vi "ATF-Disconnect RT.vi"(8 "error in (no error)":errorcluster, 10 "RT Disconnect":enum16{"Both", "Pump", "Storage"}(ring), 11 "Cluster in":T3) -> (0 "error out":errorcluster, 2 "status":string, 3 "Cluster out":T3)   [LabVIEW 2022 SP3]
uses:
  Controls/SeCrTs-boolean ref.ctl
  Controls/SeCrTs-EPV .ctl
  75c43d07-cfec-4a61-aeb0-3d2073dd9aa1.vi
  ebca87ca-1d58-4613-b13f-b88391691f9b.vi
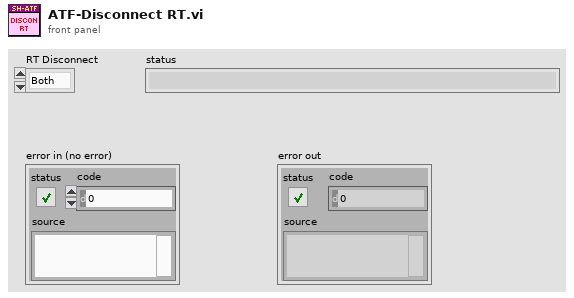
[diagram p1: front panel]
types:
  T1 = typedef "SeCrTs-boolean ref.ctl" = cluster{"Connect RT":refnum<vi>, "START DAQ":refnum<vi>, "STOP DAQ":refnum<vi>, "DAQ SETTING":refnum<vi>, "START LOG":refnum<vi>, "STOP LOG":refnum<vi>, "Connect Drive ATF":refnum<vi>, "Update drive ATF":refnum<vi>, "Gate driver ATF":refnum<vi>, "Motor On ATF":refnum<vi>, "ADC reset ATF":refnum<vi>, "Gate driver ATF 2":refnum<vi>, "Motor off ATF":refnum<vi>, "MCU reset ATF":refnum<vi>, "Connect Drive Lox":refnum<vi>, "Update drive lox":refnum<vi>, "Gate driver- LOX":refnum<vi>, "Motor On lox":refnum<vi>, "Adc reset lox":refnum<vi>, "MCU Reset -LOX":refnum<vi>, "Motor Off lox":refnum<vi>, "Connect ppsu":refnum<vi>, "update ppsu":refnum<vi>, "DC on":refnum<vi>, "Alarm ack":refnum<vi>, "DC off":refnum<vi>, "Ms initialize":refnum<vi>, "Exit RT":refnum<vi>, "ABORT":refnum<vi>, "HOLD UPDATE":refnum<vi>, "Log type":refnum<vi>, "PUMP IP":refnum<vi>, "STORAGE IP":refnum<vi>}
  T2 = typedef "SeCrTs-EPV .ctl" = cluster{"F_EPV_131":refnum<vi>, "F_EPV_132":refnum<vi>, "F_EPV_136":refnum<vi>, "F_EPV_21":refnum<vi>, "F_EPV_41":refnum<vi>, "N_EPV_68":refnum<vi>, "N_EPV_ 69":refnum<vi>, "N_EPV_ 33":refnum<vi>, "F_EPV_142":refnum<vi>, "F_EPV_28":refnum<vi>, "N_EPV_203":refnum<vi>, "N_EPV_206":refnum<vi>, "F_EPV_75":refnum<vi>, "C_EPV_2":refnum<vi>, "C_EPV_7":refnum<vi>, "C_EPV_8":refnum<vi>, "C_EPV_123":refnum<vi>, "C_EPV_124":refnum<vi>, "C_EPV_127":refnum<vi>, "N_EPV_62a":refnum<vi>, "N_EPV_62b":refnum<vi>, "N_EPV_61":refnum<vi>, "G_EPV_51":refnum<vi>, "N_EPV_141":refnum<vi>, "C_EPV_803":refnum<vi>, "C_EPV_18":refnum<vi>, "C_EPV_1352":refnum<vi>, "N_EPV_202":refnum<vi>, "C_EPV_16":refnum<vi>}
  T3 = cluster{"Bol":T1, "EPV":T2, "Covers":cluster{"cover":refnum<vi>, "Login screen cover":refnum<vi>, "cover Motor":refnum<vi>}, "Log cmd":cluster{"C/NC":bool, "Start/Stop Log":bool[], "Log Name":string, "Config":cluster{"AO config":cluster{"Channel_Name":string, "Channel_Number":string, "Default_Value":dbl, "Units":string}[], "AI config":cluster{"Channel_Name":string, "Channel_Number":string, "Pre_Scale_min":dbl, "Pre_Scale_max":dbl, "Sensor_min":dbl, "Sensor_max":dbl, "Units":string}[], "DI config":cluster{"Channel_Name":string, "Channel_Number":string, "Default_Value":bool, "DI invert?":bool}[], "DO config":cluster{"Channel_Name":string, "Channel_Number":string, "Default_Value":bool, "DO invert?":bool}[], "TC config":cluster{"Channel_Name":string, "Channel_Number":string, "Pre_Scale_min":dbl, "Pre_Scale_max":dbl, "units":i32, " type":i32}[], "ACC config":cluster{"Channel_Name":string, "Channel_Number":string, "Pre_Scale_min":dbl, "Pre_Scale_max":dbl, "Terminal configuration":i32, "Sensitivity":dbl, "Sensitivity units":i32}[], "SG config":cluster{"Channel_Name":string, "Channel_Number":string, "Pre_Scale_min":dbl, "Pre_Scale_max":dbl}[], "Strain Gauge Settings":cluster{"poisson ratio":dbl, "nominal gage resistance":dbl, "gage factor":dbl}, "Bridge Settings":cluster{"voltage excitation value":dbl, "voltage excitation source":i32, "initial bridge voltage":dbl, "lead wire resistance":dbl, "strain configuration":i32}, "Sample Rate":cluster{"AI Sample Rate":dbl[], "AO Sample Rate":dbl[], "DI Sample Rate":dbl[], "TC Sample Rate":dbl[], "DO Sample Rate":dbl[], "SG Sample Rate":dbl[], "ACC Sample Rate":dbl[]}}, "Log min":dbl}, "STORAGE IP":string, "PUMP IP":string, "Storage con":bool, "Pumb con":bool}
  T4 = enum8{"Enabled", "Disabled", "Disabled and Grayed Out"}
  T5 = enum8{"Enabled", "Disabled", "Disabled and Grayed Out"}[]
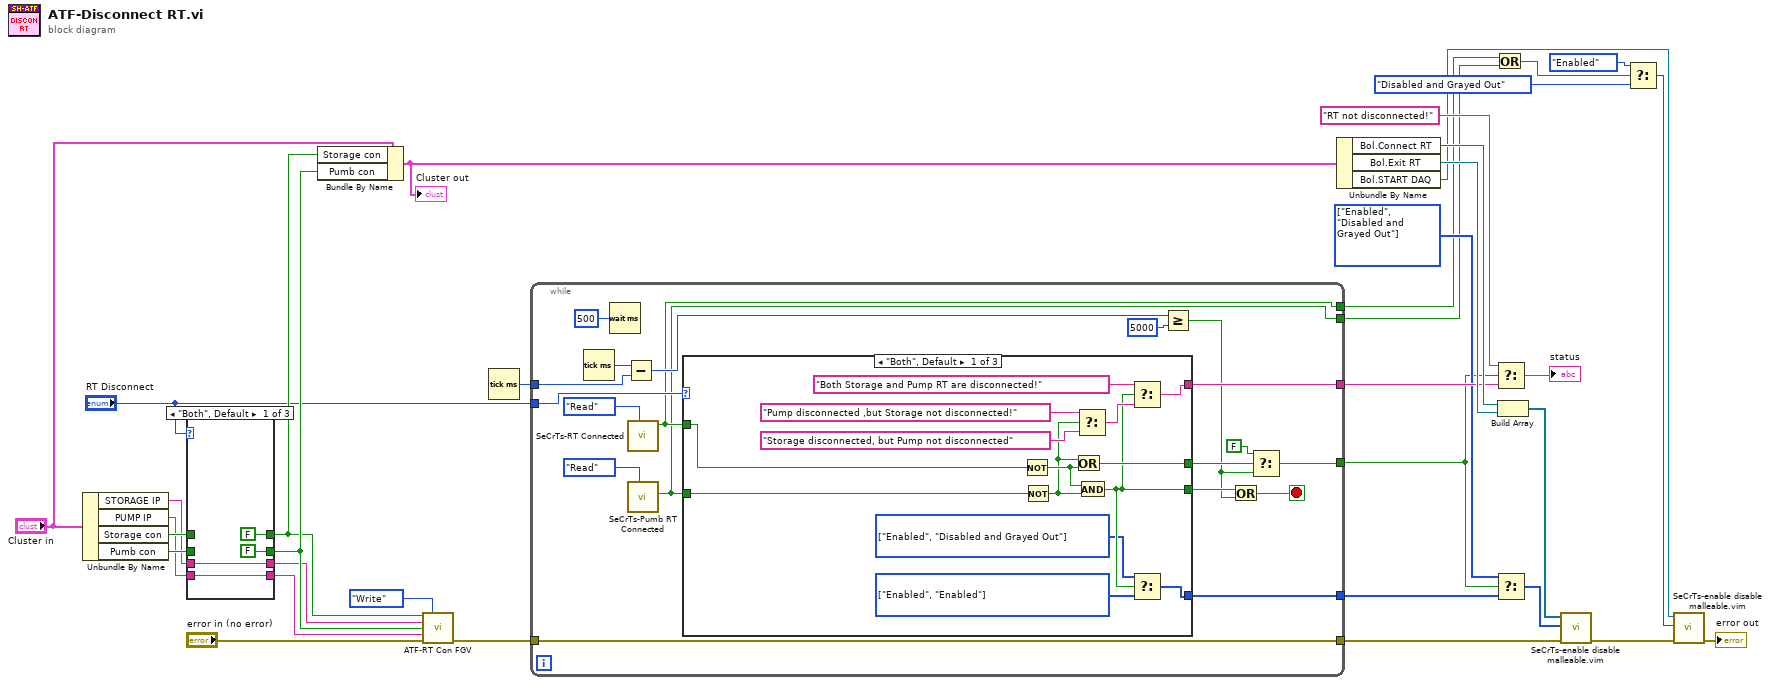
[diagram p0: block diagram]
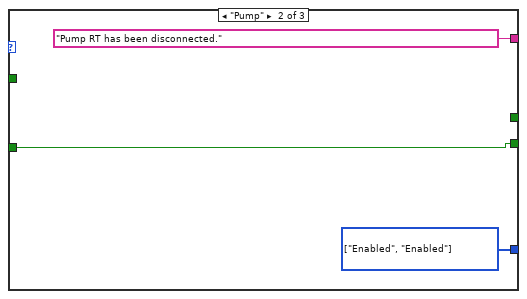
[diagram p2: hidden frame]
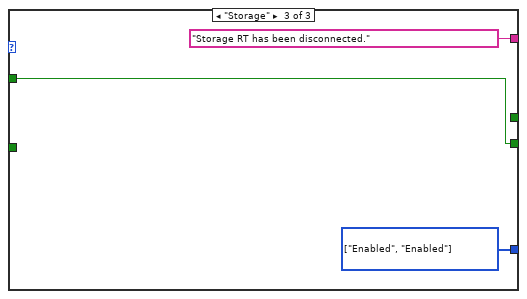
[diagram p3: hidden frame]
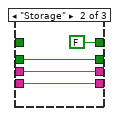
[diagram p4: hidden frame]
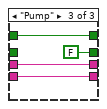
[diagram p5: hidden frame]
diagram:
  w17 = T5 [enum."Enabled", enum."Disabled and Grayed Out"] items=["Enabled", "Disabled", "Disabled and Grayed Out"] ("t")
  n1 = Unbundle By Name("Cluster in") -> ("STORAGE IP"=w30:string, "PUMP IP"=w31:string, "Storage con"=w32:bool, "Pumb con"=w33:bool)
  n2 = case shown="\"Both\", Default" "RT Disconnect" {
    tunnel: [w37 w42 w47] -> w27
    tunnel: [FALSE ("Storage rt con") FALSE ("Storage rt con") w44] -> w34
    tunnel: w30 -> [w37 w42 w47]
    tunnel: w31 -> [w36 w41 w46]
    tunnel: [w36 w41 w46] -> w29
    tunnel: [FALSE ("Pumb rt con") w40 FALSE ("Pumb rt con")] -> w35
    tunnel: w32 -> [_ _ w44]
    tunnel: w33 -> [_ w40 _]
    frame "Both", Default {
    }
    frame "Storage" {
    }
    frame "Pump" {
    }
  }
  n3 = Bundle By Name(cluster="Cluster in", "Storage con"=w34, "Pumb con"=w35) -> (w11:T3)
  "Cluster out" <- w11
  n4 = call "ATF-RT Con FGV.vi"("Storage rt con"=w34, "Enum"=enum16{"Read", "Write"}."Write", "Storage IP"=w27, "Pumb rt con"=w35, "Pump IP"=w29, "error in"="error in (no error)") -> ("error out"=w13:errorcluster)  [unwired: 5 in, 4 out]
  n5 = Tick Count (ms)() -> (millisecond timer value=w24:u32)
  n6 = while {
    tunnel: w13 -> [w66]
    tunnel: [w66] -> w15
    tunnel: w24 -> [w64]
    tunnel: "RT Disconnect" -> [w59]
    tunnel: [w56] -> w20
    tunnel: [w55] -> w19
    tunnel: [w54] -> w5
    tunnel: [w49] -> w3
    tunnel: [w48] -> w2
    stop <- w57 stop-if-true
    n7 = Tick Count (ms)() -> (millisecond timer value=w65:u32)
    n8 = Wait (ms)(milliseconds to wait=u32 500) -> ()  [unwired: 1 out]
    n9 = Subtract(x=w65, y=w64) -> (x-y=w63:u32)
    n10 = call "SeCrTs-RT Connected .vi"("Enum"=enum16{"Read", "Write"}."Read") -> ("Stoarge rt con R"=w49:bool)  [unwired: 9 in, 1 out]
    n11 = call "SeCrTs-Pumb RT Connected.vi"("Enum"=enum16{"Read", "Write"}."Read") -> ("Pumb rt con R"=w48:bool)  [unwired: 9 in, 1 out]
    n12 = case shown="\"Both\", Default" w59 {
      tunnel: w49 -> [w70 _ w86]
      tunnel: w48 -> [w68 w83 _]
      tunnel: [w74 w83 w86] -> w58
      tunnel: [w71 w82 w84] -> w56
      tunnel: [w76 "Pump RT has been disconnected." "Storage RT has been disconnected."] -> w55
      tunnel: [w75 _ _] -> w53
      frame "Both", Default {
        w72 = T5 [enum."Enabled", enum."Enabled"] items=["Enabled", "Disabled", "Disabled and Grayed Out"] ("Data out")
        w73 = T5 [enum."Enabled", enum."Disabled and Grayed Out"] items=["Enabled", "Disabled", "Disabled and Grayed Out"] ("Data out")
        n13 = Not(x=w70) -> (.not. x?=w69:bool)
        n14 = Not(x=w68) -> (.not. x?=w67:bool)
        n15 = Or(x=w67, y=w69) -> (x .or. y?=w75:bool)
        n16 = Select(t="Pump disconnected ,but Storage not disconnected!", s=w67, f="Storage disconnected, but Pump not disconnected") -> (s? t:f=w79:string)
        n17 = And(x=w69, y=w67) -> (x .and. y?=w74:bool)
        n18 = Select(t="Both Storage and Pump RT are disconnected!", s=w74, f=w79) -> (s? t:f=w76:string)
        n19 = Select(t=w73, s=w74, f=w72) -> (s? t:f=w71:T5)
      }
      frame "Pump" {
        w82 = T5 [enum."Enabled", enum."Enabled"] items=["Enabled", "Disabled", "Disabled and Grayed Out"] ("Data out")
      }
      frame "Storage" {
        w84 = T5 [enum."Enabled", enum."Enabled"] items=["Enabled", "Disabled", "Disabled and Grayed Out"] ("Data out")
      }
    }
    n20 = Greater Or Equal?(x=w63, y=u32 5000) -> (x >= y?=w51:bool)
    n21 = Or(x=w58, y=w51) -> (x .or. y?=w57:bool)
    n22 = Select(t=FALSE, s=w53, f=w51) -> (s? t:f=w54:bool)
  }
  n23 = Unbundle By Name(w11) -> ("Bol.Connect RT"=w23:refnum<vi>, "Bol.Exit RT"=w22:refnum<vi>, "Bol.START DAQ"=w8:refnum<vi>)
  n24 = Or(x=w3, y=w2) -> (x .or. y?=w1:bool)
  n25 = Select(t="RT not disconnected!", s=w5, f=w19) -> (s? t:f=→"status":string)
  n26 = Select(t=w17, s=w5, f=w20) -> (s? t:f=w16:T5)
  n27 = Build Array(w23, w22) -> (w21:refnum<vi>[])
  n28 = call "SeCrTs-enable disable malleable.vim"("error in"=w15, "Data"=w16, "Ref in"=w21) -> ("error out"=w10:errorcluster)  [unwired: 7 in, 1 out]
  n29 = Select(t=T4."Enabled" ("Disabled"), s=w1, f=T4."Disabled and Grayed Out" ("Disabled")) -> (s? t:f=w4:T4)
  n30 = call "SeCrTs-enable disable malleable.vim"("error in"=w10, "Data"=w4, "Ref in"=w8) -> ("error out"=→"error out":errorcluster)  [unwired: 7 in, 1 out]
